vi "Helm Heading PID Cycle TEST.vi"() -> ()   [LabVIEW 2015]
uses:
  <vilib>/addons/control/pid/NI_PID_pid.lvlib
  <vilib>/addons/control/pid/pid.llb/PID (DBL).vi
panel:
  in  "Close":bool
  in  "Reset Plant":bool
  in  "stop":bool
  in  "Sampling Rate":dbl=30.0
  out "Process variable and Setpoint":cluster{"initial PV":dbl, "SP:":dbl}(graph)
  in  "PID gains":T1={"proportional gain (Kc)"=1.0, "integral time (Ti, min)"=0.01, "derivative time (Td, min)"=0.0} {"derivative time (Td, min)" format="%#_11f"; "integral time (Ti, min)" format="%#.9f"; "proportional gain (Kc)" format="%.3f"}
  in  "Gauge":cluster{dbl, dbl}(knob)={0.0, 16.871828399534785} scale=0.0..360.0
  out "Rudder Command":dbl(graph)
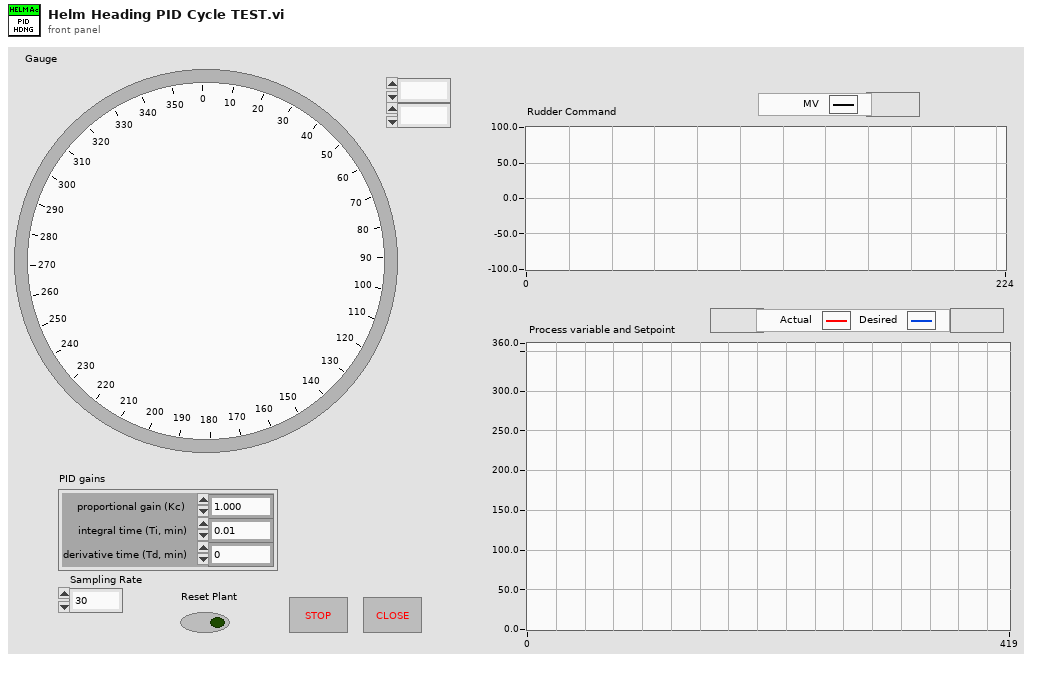
[diagram p1: front panel]
types:
  T1 = cluster{"proportional gain (Kc)":dbl, "integral time (Ti, min)":dbl, "derivative time (Td, min)":dbl}
  T2 = cluster{"static gain":dbl, "lag (min)":dbl, "dead cycles":dbl, "load %":dbl, "deadband":dbl, "noise level %":dbl, "initial PV":dbl, "initial PV 2":dbl}
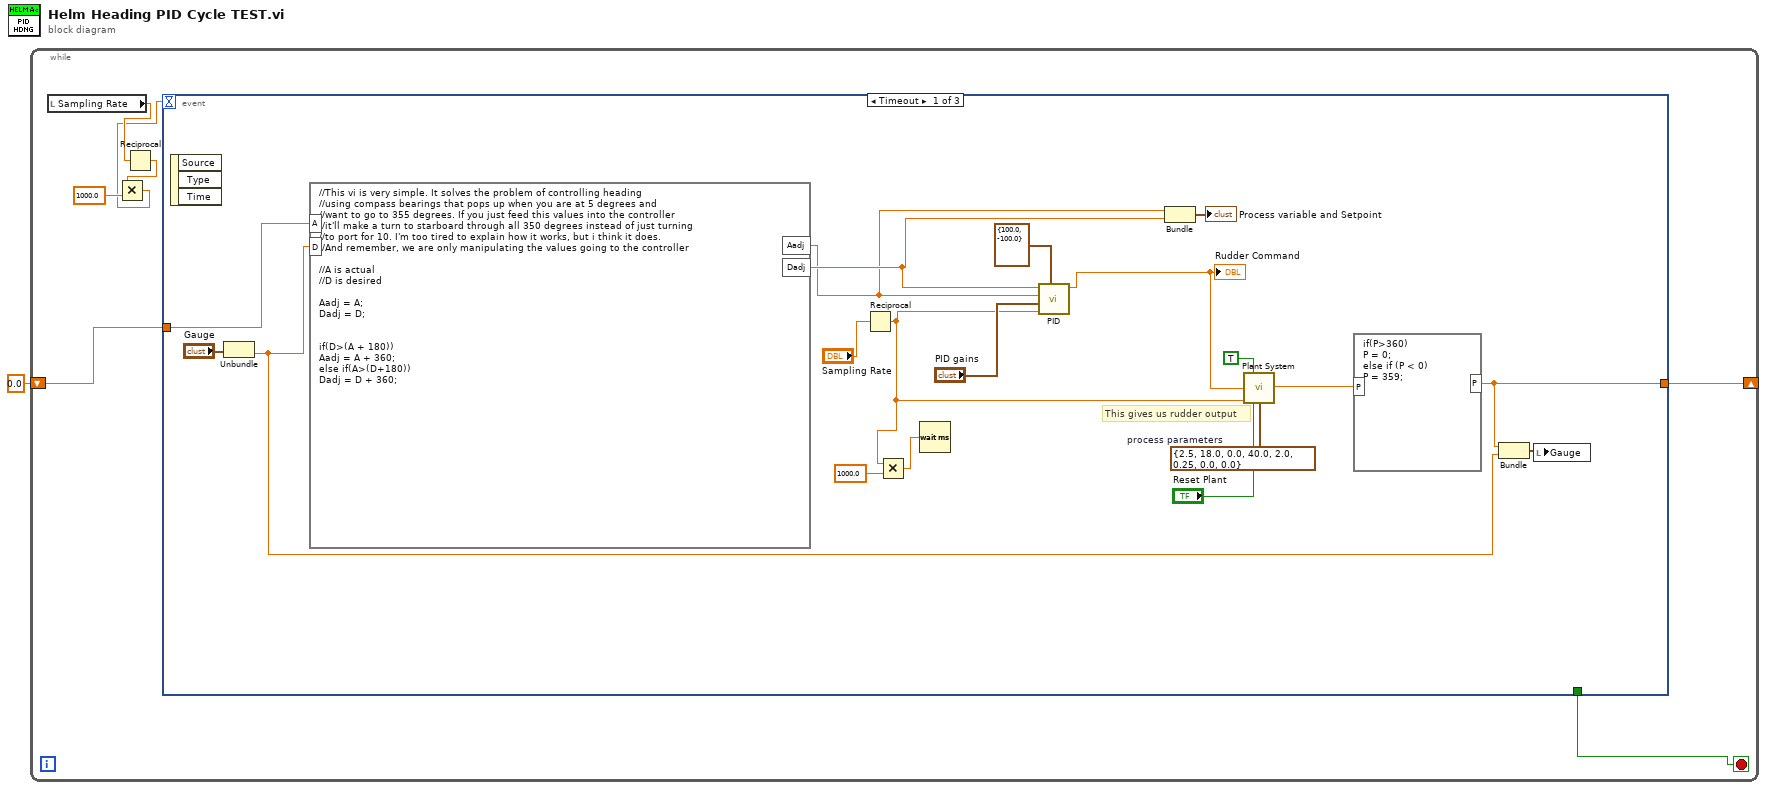
[diagram p0: block diagram]
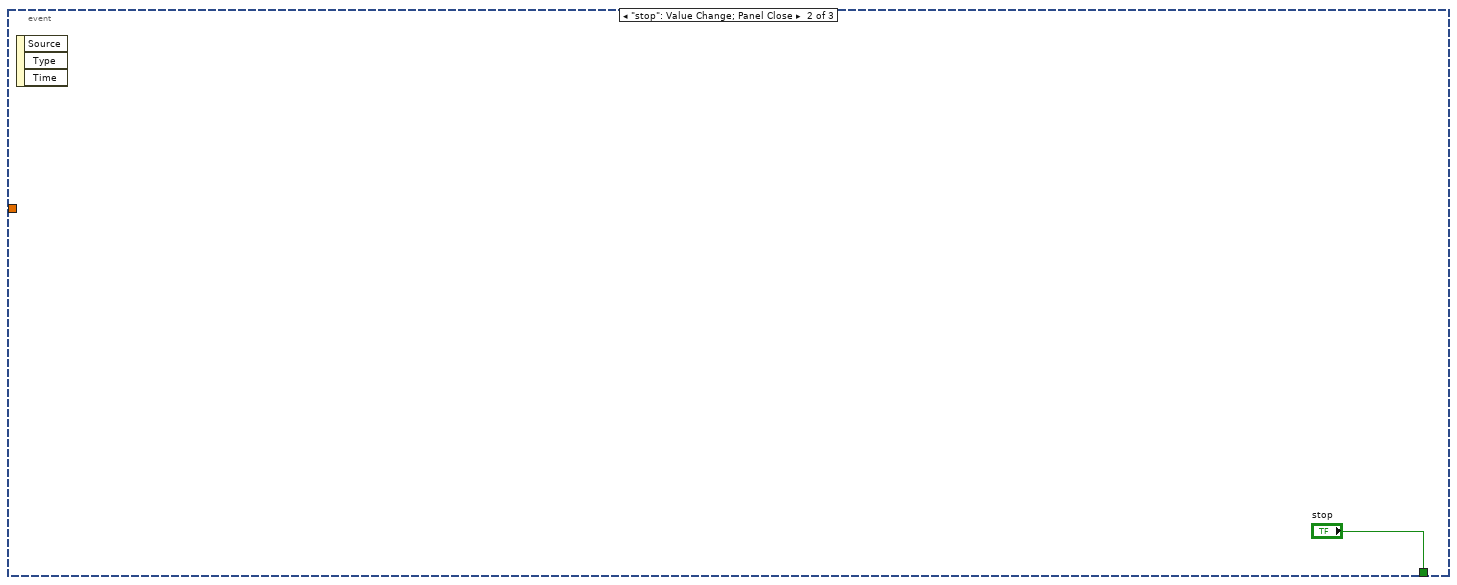
[diagram p2: hidden frame]
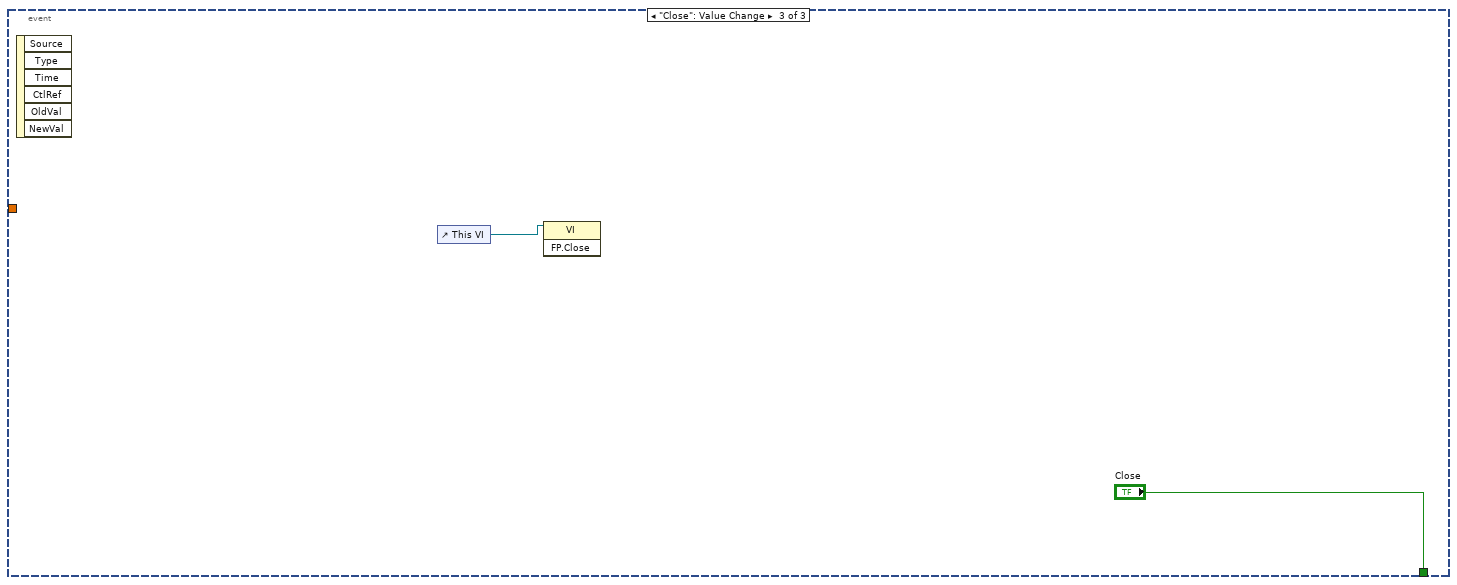
[diagram p3: hidden frame]
diagram:
  n1 = while {
    shift-right: [w8] -> _
    shift-left: 0.0 ("P") -> [w7]
    stop <- w6 stop-if-true
    n2 = local read "Sampling Rate"() -> (w5:dbl)
    n3 = Reciprocal(x=w5) -> (1/x=w3:dbl)
    n4 = Multiply(x=w3, y=1000.0) -> (x*y=w2:dbl)
    n5 = event shown="[0] Timeout" {
      selector: _ -> [_ _ _]
      dyn-events: _ -> [_ _ _]
      timeout: w2 -> [_ _ _]
      tunnel: w7 -> [w27 _ _]
      tunnel: [w9 _ _] -> w8
      tunnel: [_ "stop" "Close"] -> w6
      event Timeout {
        w22 = T2 {"static gain"=2.5, "lag (min)"=18.0, "dead cycles"=0.0, "load %"=40.0, "deadband"=2.0, "noise level %"=0.25, "initial PV"=0.0, "initial PV 2"=0.0}  # process parameters
        # "This gives us rudder output"
        n6 = event-data() -> ()  [unwired: 1 in, 3 out]
        n7 = Unbundle("Gauge") -> (w11:dbl)  [unwired: 1 out]
        n8 = formula code="//This vi is very simple. It solves the problem of controlling heading\n//using compass bearings that pops up when you are at 5 degrees and\n//want to go to 355 degrees. If you just feed this values into the controller\n//it'll make a turn to starboard through all 350 degrees instead of just turning\n//to port for 10. I'm too tired to explain how it works, but i think it does.\n//And remember, we are only manipulating the values going to the controller\n\n//A is actual\n//D is desired\n\nAadj = A;\nDadj = D;\n\n\nif(D>(A + 180))\nAadj = A + 360;\nelse if(A>(D+180))\nDadj = D + 360;"("A"=w27, "D"=w11) -> ("Aadj"=w17:dbl, "Dadj"=w18:dbl)
        n9 = Reciprocal(x="Sampling Rate") -> (1/x=w16:dbl)
        n10 = Multiply(x=w16, y=1000.0) -> (x*y=w14:dbl)
        n11 = Wait (ms)(milliseconds to wait=w14) -> ()  [unwired: 1 out]
        n12 = call-poly <vilib>:"PID.vi"("output range"=cluster{"output high":dbl, "output low":dbl} {"output high"=100.0, "output low"=-100.0}, "dt (s)"=w16, "PID gains"="PID gains", "process variable"=w17, "setpoint"=w18) -> ("output"=w19:dbl)  [unwired: 5 in, 1 out]
        "Rudder Command" <- w19
        n13 = Bundle("Aadj"=w17, "Dadj"=w18) -> (→"Process variable and Setpoint":cluster{"Aadj":dbl, "Dadj":dbl})  [unwired: 1 in]
        n14 = call "Plant System.vi"("Integrator ?"=TRUE, "Plant Input"=w19, "dt (s)"=w16, "reinitialize? (F)"="Reset Plant", "process parameters"=w22) -> ("Plant Output"=w13:dbl)  [unwired: 10 in]
        n15 = formula code="if(P>360)\nP = 0;\nelse if (P < 0)\nP = 359;"("P"=w13) -> ("P"=w9:dbl)
        n16 = Bundle("P"=w9, w11) -> (w12:cluster{"P":dbl, dbl})  [unwired: 1 in]
        n17 = local write "Gauge"(w12) -> ()
      }
      event "stop": Value Change; Panel Close {
        n18 = event-data() -> ()  [unwired: 1 in, 3 out]
      }
      event "Close": Value Change {
        n19 = event-data() -> ()  [unwired: 1 in, 6 out]
        n20 = control-ref of="This VI"() -> (w29:refnum<vi>)
        n21 = invoke class="VI" method="FP.Close"(reference=w29) -> ()  [unwired: 2 in, 3 out]
      }
    }
  }
